vi "ExerciseE1.7.vi"() -> ()   [LabVIEW 2018]
panel:
  out "I":dbl
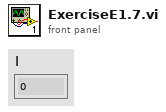
[diagram p1: front panel]
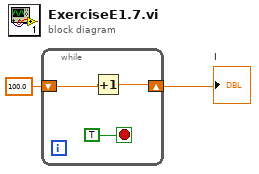
[diagram p0: block diagram]
diagram:
  n1 = while {
    shift-right: [w3] -> w2
    shift-left: 100.0 -> [w4]
    stop <- TRUE stop-if-true
    n2 = Increment(x=w4) -> (x+1=w3:dbl)
  }
  "I" <- w2
